vi "Windows.SetAlwaysOnTop.vi"(8 "error in (no error)":errorcluster, 10 "Window Name (\"\")":string) -> (0 "error out":errorcluster, 2 "success?":bool)   [LabVIEW 2019, in "Tools.lvlib"]
doc: "This function will make the window Always on Top. Window Name is Window Title from Title Bar, not application name!"
uses:
  Tools.lvlib
  user32.dll
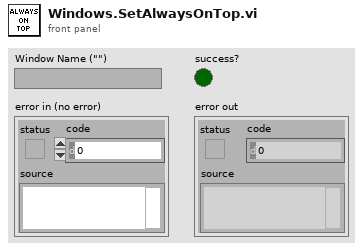
[diagram p1: front panel]
types:
  T1 = cluster{"RECT[0]":i32, "RECT[1]":i32, "RECT[2]":i32, "RECT[3]":i32}
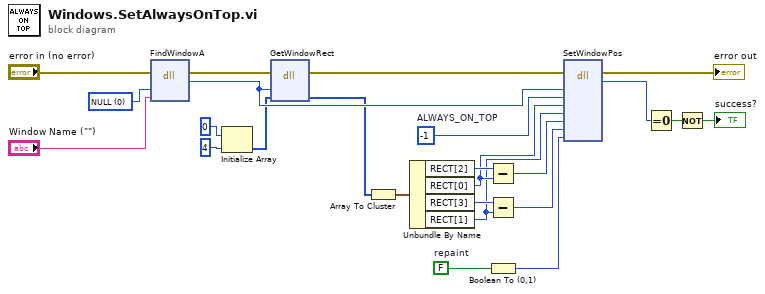
[diagram p0: block diagram]
diagram:
  w12 = 0 items=["NULL"]
  w15 = -1  # ALWAYS_ON_TOP
  w19 = FALSE  # repaint
  n1 = dll-call lib="user32.dll" fn="FindWindowA" label="FindWindow"(error in="error in (no error)", "lpszClassName"=w12, "lpszWindowName"="Window Name (\"\")") -> (error out=w21:errorcluster, "hWnd"=w11:u32)  [unwired: 4 in, 1 out]
  n2 = Initialize Array(0, 4) -> (w9:i32[])
  n3 = dll-call lib="USER32.DLL" fn="GetWindowRect"(error in=w21, "hWnd"=w11, "RECT"=w9) -> (error out=w20:errorcluster, "RECT"=w10:i32[])  [unwired: 3 in, 2 out]
  n4 = Array To Cluster(array=w10) -> (cluster=w24:T1)
  n5 = Unbundle By Name(w24) -> ("RECT[2]"=w5:i32, "RECT[0]"=w4:i32, "RECT[3]"=w6:i32, "RECT[1]"=w3:i32)
  n6 = Subtract(x=w5, y=w4) -> (x-y=w2:i32)
  n7 = Subtract(x=w6, y=w3) -> (x-y=w1:i32)
  n8 = Boolean To (0,1)(Boolean=w19) -> (0, 1=w18:i16)
  n9 = dll-call lib="USER32.DLL" fn="SetWindowPos" label="MoveWindow"(error in=w20, "hWnd"=w11, "hWndInsertAfter"=w15, "left"=w4, "top"=w3, "right"=w2, "bottom"=w1, "repaint"=w18) -> (error out=→"error out":errorcluster, "error"=w17:i32)  [unwired: 4 in, 6 out]
  n10 = Equal To 0?(x=w17) -> (x = 0?=w16:bool)
  n11 = Not(x=w16) -> (.not. x?=→"success?":bool)
